vi "Calculate Wfm Subset for Measurement.vi"(6 "sampling rate":dbl, 7 "signal frequency":dbl, 8 "minimum settling duration":dbl, 9 "minimum settling cycles":u32, 10 "minimum measurement duration":dbl, 11 "minimum measurement cycles":u32) -> (1 "total acquisition (samples)":u32, 2 "duration (samples)":u32, 3 "start (samples)":u32)   [LabVIEW 2021]
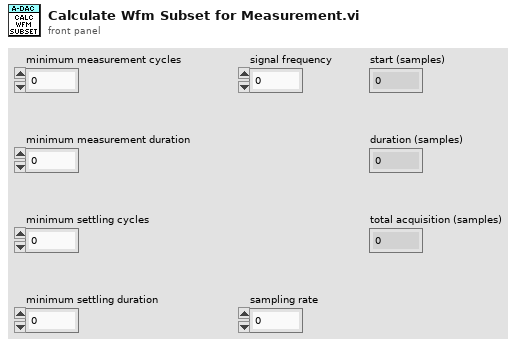
[diagram p1: front panel]
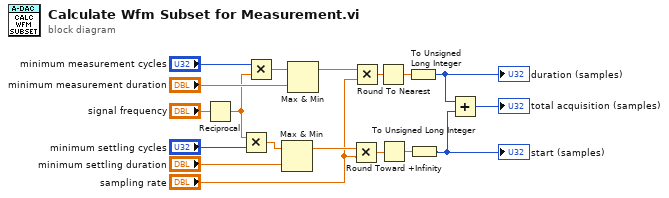
[diagram p0: block diagram]
diagram:
  n1 = Reciprocal(x="signal frequency") -> (1/x=w1:dbl)
  n2 = Multiply(x=w1, y="minimum settling cycles") -> (x*y=w15:dbl)
  n3 = Multiply(x="minimum measurement cycles", y=w1) -> (x*y=w17:dbl)
  n4 = Max & Min(x=w15, y="minimum settling duration") -> (max(x,y)=w14:dbl)  [unwired: 1 out]
  n5 = Max & Min(x=w17, y="minimum measurement duration") -> (max(x,y)=w13:dbl)  [unwired: 1 out]
  n6 = Multiply(x=w14, y="sampling rate") -> (x*y=w8:dbl)
  n7 = Multiply(x=w13, y="sampling rate") -> (x*y=w4:dbl)
  n8 = Round To Nearest(number=w4) -> (nearest integer value=w5:dbl)
  n9 = Round Toward +Infinity(x=w8) -> (ceil(x): smallest int >= x=w7:dbl)
  n10 = To Unsigned Long Integer(number=w5) -> (unsigned 32bit integer=w3:u32)
  "duration (samples)" <- w3
  n11 = To Unsigned Long Integer(number=w7) -> (unsigned 32bit integer=w6:u32)
  "start (samples)" <- w6
  n12 = Add(x=w3, y=w6) -> (x+y=→"total acquisition (samples)":u32)
